vi "ADCP_Remote_Request_Frames.vi"(8 "error in (no error)":errorcluster, 9 "Request Frame IDs":u8[](array[numeric]), 10 "Node ID":i32=-1, 11 "ADCP In":refnum<class "ADCP.lvclass">) -> (0 "error out":errorcluster, 1 "Error and Status":T1, 2 "Remote Request":T2, 3 "ADCP Out":refnum<class "ADCP.lvclass">)   [LabVIEW 2017, in "ADCP.lvclass"]
uses:
  ADCP.lvclass
  ADCP.lvclass/ADCP.ctl
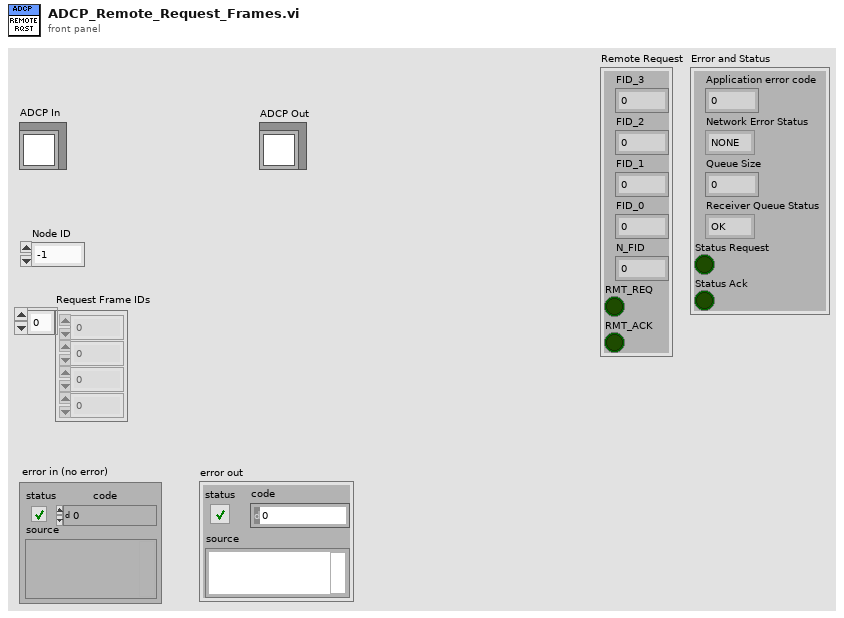
[diagram p1: front panel]
types:
  T1 = cluster{"Application error code":u16, "Network Error Status":enum16{"NONE", "CONNECTION_ALREADY_OPEN", "CONNECTION_ALREADY_CLOSED", "INVALID_FRAME_REQUEST"}, "Queue Size":u16, "Receiver Queue Status":enum16{"OK", "EMPTY", "FULL"}, "Status Request":bool, "Status Ack":bool}
  T2 = cluster{"FID_3":u8, "FID_2":u8, "FID_1":u8, "FID_0":u8, "N_FID":u8, "RMT_REQ":bool, "RMT_ACK":bool}
  T3 = typedef "ADCP.lvclass/ADCP_Packet_Info.ctl" = cluster{"Priority":enum16{"LOW", "HIGH"}, "Type":enum16{"Data", "Connection Management", "Remote Request", "Error and status", "INVALID"}, "Node ID":i32, "Frame ID":i32, "Checksum valid ?":bool, "Current time (ms)":u32}
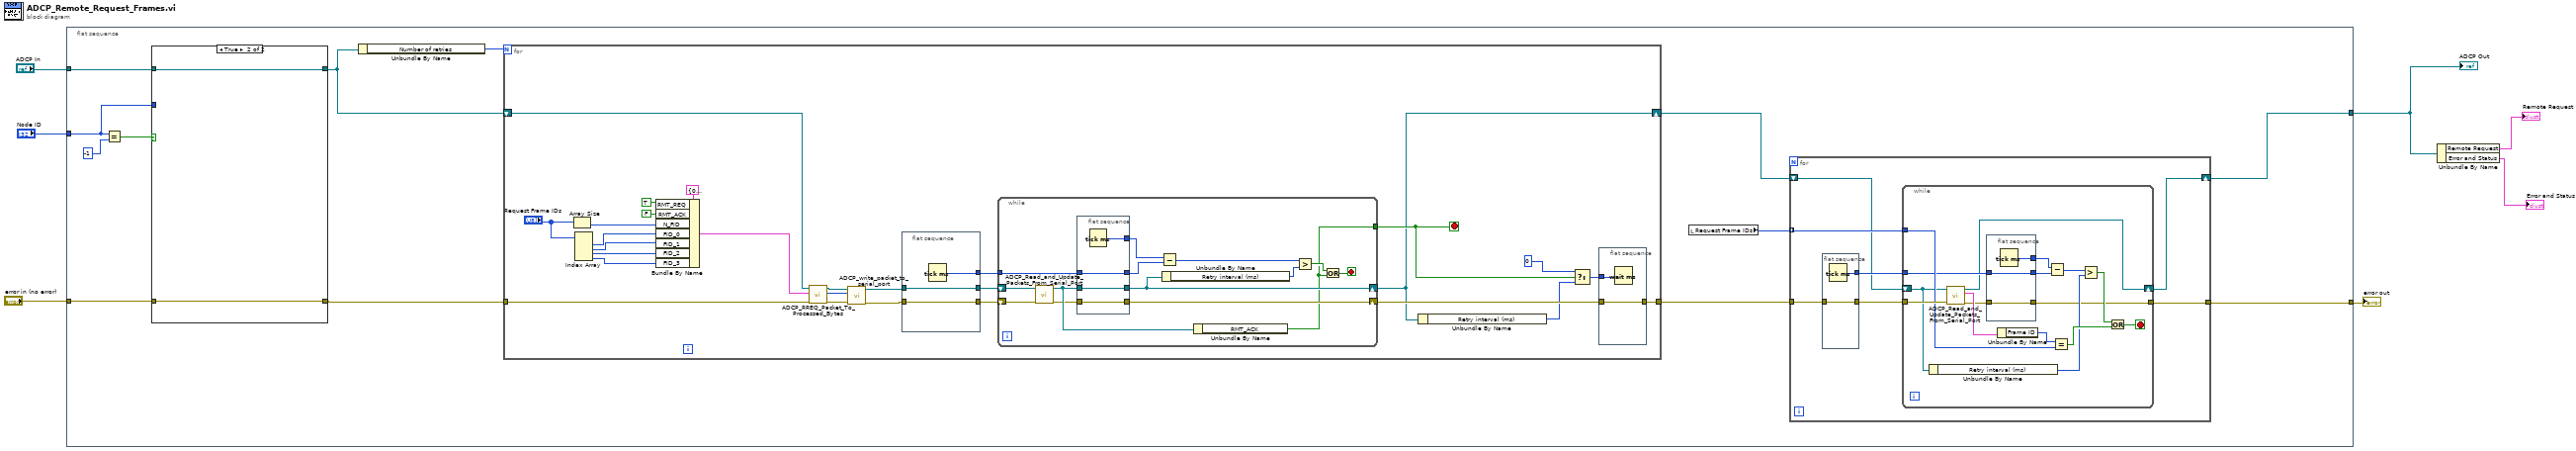
[diagram p0: block diagram]
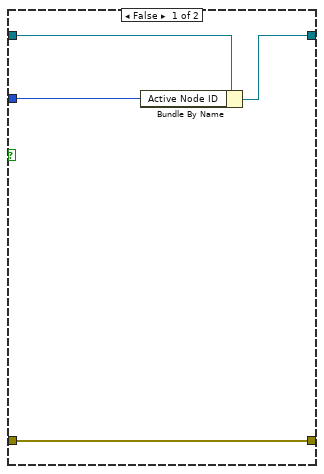
[diagram p2: hidden frame]
diagram:
  n1 = flat-sequence {
    tunnel: "ADCP In" -> [w17]
    tunnel: "error in (no error)" -> [w19]
    tunnel: "Node ID" -> [w16]
    tunnel: [w8] -> w3
    tunnel: [w10] -> w4
    frame #0 {
      n2 = Equal?(x=w16, y=-1) -> (x = y?=w18:bool)
      n3 = case shown="True" w18 {
        tunnel: w19 -> [w99 w103]
        tunnel: w17 -> [w102 w104]
        tunnel: [w100 w104] -> w13
        tunnel: w16 -> [w101 _]
        tunnel: [w99 w103] -> w15
        frame False {
          n4 = Bundle By Name(cluster=w102, "Active Node ID"=w101) -> (w100:refnum<class "ADCP.lvclass">)
        }
        frame True {
        }
      }
      n5 = Unbundle By Name(w13) -> ("Number of retries"=w14:u16)
      n6 = for {
        N: w14 -> [_]
        tunnel: w15 -> [w75]
        shift-right: [w66] -> w9
        shift-left: w13 -> [w74]
        tunnel: [w64] -> w12
        stop <- w69 stop-if-true
        n7 = Array Size(array="Request Frame IDs") -> (size(s)=w55:i32)
        n8 = Index Array(array="Request Frame IDs") -> (element #1=w53:u8, element #2=w52:u8, element #3=w51:u8, element #4=w50:u8)  [unwired: 4 in]
        n9 = Bundle By Name(cluster=T2 {"FID_3"=0, "FID_2"=0, "FID_1"=0, "FID_0"=0, "N_FID"=0, "RMT_REQ"=FALSE, "RMT_ACK"=FALSE} ("RREQ_Packet"), "RMT_REQ"=TRUE, "RMT_ACK"=FALSE, "N_FID"=w55, "FID_0"=w53, "FID_1"=w52, "FID_2"=w51, "FID_3"=w50) -> (w49:T2)
        n10 = call "ADCP_RREQ_Packet_To_Processed_Bytes.vi"("error in (no error)"=w75, "RREQ_Packet"=w49, "ADCP In"=w74) -> ("error out"=w61:errorcluster, "Processed Packet Bytes"=w63:u8[], "ADCP Out"=w62:refnum<class "ADCP.lvclass">)  [unwired: 6 in]
        n11 = call "ADCP_write_packet_to_serial_port.vi"("error in (no error)"=w61, "Packet Bytes"=w63, "ADCP In"=w62) -> ("error out"=w60:errorcluster, "ADCP Out"=w59:refnum<class "ADCP.lvclass">)  [unwired: 7 in]
        n12 = flat-sequence {
          tunnel: w59 -> [w80]
          tunnel: [w80] -> w73
          tunnel: w60 -> [w79]
          tunnel: [w79] -> w72
          tunnel: [w78] -> w71
          frame #0 {
            n13 = Tick Count (ms)() -> (millisecond timer value=w78:u32)
          }
        }
        n14 = while {
          shift-right: [w85] -> w66
          shift-left: w73 -> [w93]
          shift-right: [w90] -> w70
          shift-left: w72 -> [w94]
          tunnel: w71 -> [w88]
          tunnel: [w81] -> w69
          stop <- w82 stop-if-true
          n15 = call "ADCP_Read_and_Update_Packets_From_Serial_Port.vi"("error in (no error)"=w94, "ADCP In"=w93) -> ("error out"=w91:errorcluster, "ADCP out"=w92:refnum<class "ADCP.lvclass">)  [unwired: 6 in, 2 out]
          n16 = flat-sequence {
            tunnel: w92 -> [w98]
            tunnel: [w98] -> w85
            tunnel: w91 -> [w97]
            tunnel: [w97] -> w90
            tunnel: [w96] -> w89
            tunnel: w88 -> [w95]
            tunnel: [w95] -> w87
            frame #0 {
              n17 = Tick Count (ms)() -> (millisecond timer value=w96:u32)
            }
          }
          n18 = Subtract(x=w89, y=w87) -> (x-y=w86:u32)
          n19 = Unbundle By Name(w85) -> ("Retry interval (ms)"=w84:u16)
          n20 = Unbundle By Name(w92) -> ("RMT_ACK"=w81:bool)
          n21 = Greater?(x=w86, y=w84) -> (0:w83:bool)
          n22 = Or(x=w83, y=w81) -> (x .or. y?=w82:bool)
        }
        n23 = Unbundle By Name(w66) -> ("Retry interval (ms)"=w65:u16)
        n24 = Select(t=0, s=w69, f=w65) -> (s? t:f=w67:i32)
        n25 = flat-sequence {
          tunnel: w70 -> [w77]
          tunnel: [w77] -> w64
          tunnel: w67 -> [w76]
          frame #0 {
            n26 = Wait (ms)(milliseconds to wait=w76) -> ()  [unwired: 1 out]
          }
        }
      }
      n27 = local read "Request Frame IDs"() -> (w11:u8[])
      n28 = for {
        tunnel: w12 -> [w27]
        tunnel: w11 -> [w24] mode=indexing
        tunnel: [w23] -> w10
        shift-right: [w21] -> w8
        shift-left: w9 -> [w22]
        n29 = flat-sequence {
          tunnel: w27 -> [w29]
          tunnel: [w29] -> w26
          tunnel: [w28] -> w25
          frame #0 {
            n30 = Tick Count (ms)() -> (millisecond timer value=w28:u32)
          }
        }
        n31 = while {
          tunnel: w26 -> [w45]
          shift-right: [w31] -> w21
          shift-left: w22 -> [w35]
          tunnel: w25 -> [w38]
          tunnel: w24 -> [w42]
          tunnel: [w32] -> w23
          stop <- w30 stop-if-true
          n32 = Unbundle By Name(w35) -> ("Retry interval (ms)"=w34:u16)
          n33 = call "ADCP_Read_and_Update_Packets_From_Serial_Port.vi"("error in (no error)"=w45, "ADCP In"=w35) -> ("error out"=w40:errorcluster, "Packet Info"=w44:T3, "ADCP out"=w31:refnum<class "ADCP.lvclass">)  [unwired: 6 in, 1 out]
          n34 = flat-sequence {
            tunnel: w40 -> [w48]
            tunnel: [w48] -> w32
            tunnel: [w47] -> w39
            tunnel: w38 -> [w46]
            tunnel: [w46] -> w37
            frame #0 {
              n35 = Tick Count (ms)() -> (millisecond timer value=w47:u32)
            }
          }
          n36 = Unbundle By Name(w44) -> ("Frame ID"=w43:i32)
          n37 = Subtract(x=w39, y=w37) -> (x-y=w36:u32)
          n38 = Equal?(x=w43, y=w42) -> (x = y?=w41:bool)
          n39 = Greater?(x=w36, y=w34) -> (0:w33:bool)
          n40 = Or(x=w33, y=w41) -> (x .or. y?=w30:bool)
        }
      }
    }
  }
  n41 = Unbundle By Name(w3) -> ("Remote Request"=→"Remote Request":T2, "Error and Status"=→"Error and Status":T1)
  "ADCP Out" <- w3
  "error out" <- w4
